vi "GenerationConfig.vi"(8 "error in (no error)":errorcluster, 11 "GenerationConfig":T2={"ExternalAtt"=0.0, "Freq"=5180000000.0, "RxPwr"=-40.0, "PacketNumber"=100, "WaveformName(WithType)"="ac80mcs9.tdms", "PhyPort"=enum."Port5"} {"RxPwr" format="%#_13g"; "Freq" format="%#_13g"; "ExternalAtt" format="%#_13g"}) -> (0 "error out":errorcluster, 3 "GenerationConfigCMD":string[](array[string])=["SOUR:RFSG:GPRF:EATTenuation 0", "SOUR:RFSG:GPRF:FREQ 5180000000", "SOUR:RFSG:GPRF:LEVel -40", "SOUR:RFSG:GPRF:PORT 'Port5'", "SOUR:RFSG:GPRF:ARB:CYCL 100", "SOUR:RFSG:GPRF:ARB:REP FINITE", "SOUR:RFSG:GPRF:ARB:WAV 'ac80mcs9.tdms'", "SOUR:RFSG:GPRF:MODE  ARB", "*OPC?"])   [LabVIEW 2015]
uses:
  PhyPort.ctl
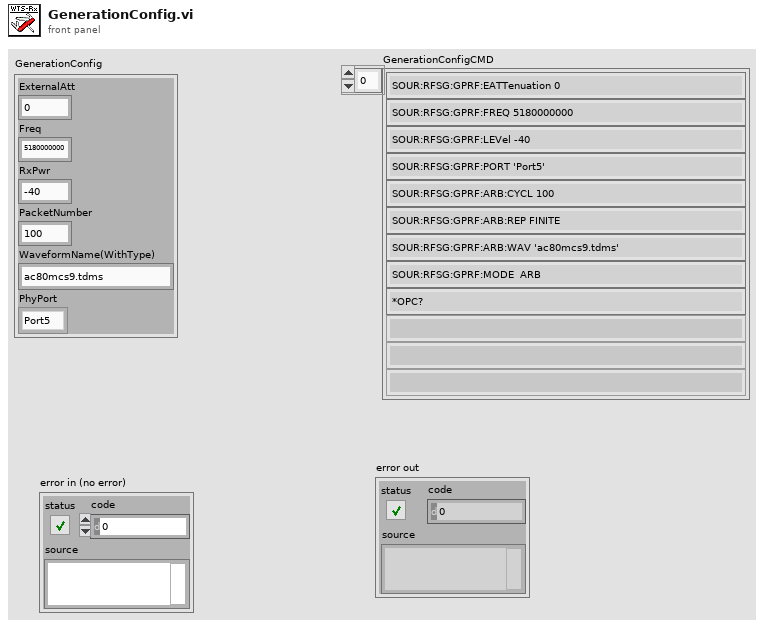
[diagram p1: front panel]
types:
  T1 = typedef "PhyPort.ctl" = enum16{"Port0", "Port1", "Port2", "Port3", "Port4", "Port5", "Port6", "Port7"}
  T2 = cluster{"ExternalAtt":dbl, "Freq":dbl, "RxPwr":dbl, "PacketNumber":i32, "WaveformName(WithType)":string, "PhyPort":T1}
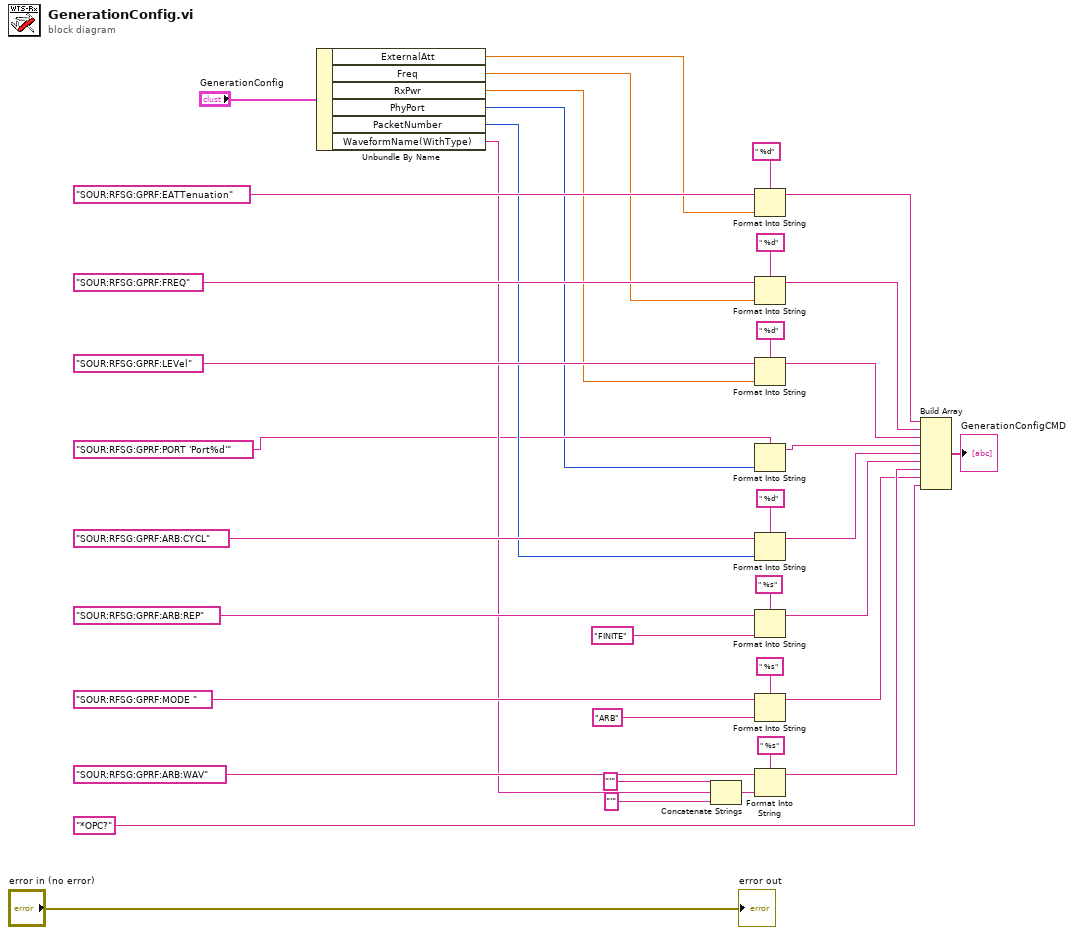
[diagram p0: block diagram]
diagram:
  n1 = Unbundle By Name("GenerationConfig") -> ("ExternalAtt"=w8:dbl, "Freq"=w7:dbl, "RxPwr"=w6:dbl, "PhyPort"=w1:T1, "PacketNumber"=w5:i32, "WaveformName(WithType)"=w4:string)
  n2 = Concatenate Strings("'", w4, "'" ("string")) -> (w22:string)
  n3 = Format Into String(format string=" %d", initial string="SOUR:RFSG:GPRF:EATTenuation", w8) -> (resulting string=w21:string)  [unwired: 1 in, 1 out]
  n4 = Format Into String(format string=" %d", initial string="SOUR:RFSG:GPRF:FREQ", w7) -> (resulting string=w20:string)  [unwired: 1 in, 1 out]
  n5 = Format Into String(format string=" %d", initial string="SOUR:RFSG:GPRF:LEVel", w6) -> (resulting string=w19:string)  [unwired: 1 in, 1 out]
  n6 = Format Into String(format string="SOUR:RFSG:GPRF:PORT 'Port%d'" ("initial string"), w1) -> (resulting string=w18:string)  [unwired: 2 in, 1 out]
  n7 = Format Into String(format string=" %d", initial string="SOUR:RFSG:GPRF:ARB:CYCL", w5) -> (resulting string=w17:string)  [unwired: 1 in, 1 out]
  n8 = Format Into String(format string=" %s", initial string="SOUR:RFSG:GPRF:ARB:REP", "FINITE" ("input 1")) -> (resulting string=w16:string)  [unwired: 1 in, 1 out]
  n9 = Format Into String(format string=" %s", initial string="SOUR:RFSG:GPRF:MODE ", "ARB" ("input 1")) -> (resulting string=w14:string)  [unwired: 1 in, 1 out]
  n10 = Format Into String(format string=" %s", initial string="SOUR:RFSG:GPRF:ARB:WAV", w22) -> (resulting string=w15:string)  [unwired: 1 in, 1 out]
  n11 = Build Array(w21, w20, w19, w18, w17, w16, w15, w14, "*OPC?") -> (→"GenerationConfigCMD":string[])
  "error out" <- "error in (no error)"
